vi "Speed Tests 2020-04-08.vi"() -> ()   [LabVIEW 2016]
uses:
  src/Data.ITX/Data.ITX.lvclass
panel:
  in  "Path":path=path "C:/temp"
  out "Another File Size":cluster{i32[], dbl[]}[](graph)=[{[0, 1, 2, 3, 4], [37.234652, 38.890539, 13.243471, 13.252304, 0.0]}, {[0, 1, 2, 3, 4], [37.234652, 38.890539, 13.243471, 13.252304, 0.0]}, {[0, 1, 2, 3, 4], [37.234652, 38.890539, 13.243471, 13.252304, 0.0]}, {[0, 1, 2, 3, 4], [37.234652, 38.890539, 13.243471, 13.252304, 0.0]}, {[0, 1, 2, 3, 4], [37.234652, 38.890539, 13.243471, 13.252304, 0.0]}, {[0, 1, 2, 3, 4], [37.234652, 38.890539, 13.243471, 13.252304, 0.0]}, {[0, 1, 2, 3, 4], [37.234652, 38.890539, 13.243471, 13.252304, 0.0]}, {[0, 1, 2, 3, 4], [37.234652, 38.890539, 13.243471, 13.252304, 0.0]}, {[0, 1, 2, 3, 4], [37.234652, 38.890539, 13.243471, 13.252304, 0.0]}, {[0, 1, 2, 3, 4], [37.234652, 38.890539, 13.243471, 13.252304, 0.0]}, {[0, 1, 2, 3, 4], [37.234652, 38.890539, 13.243471, 13.252304, 0.0]}, {[0, 1, 2, 3, 4], [37.234652, 38.890539, 13.243471, 13.252304, 0.0]}, {[0, 1, 2, 3, 4], [37.234652, 38.890539, 13.243471, 13.252304, 0.0]}, {[0, 1, 2, 3, 4], [37.234652, 38.890539, 13.243471, 13.252304, 0.0]}, {[0, 1, 2, 3, 4], [37.234652, 38.890539, 13.243471, 13.252304, 0.0]}, {[0, 1, 2, 3, 4], [37.234652, 38.890539, 13.243471, 13.252304, 0.0]}, {[0, 1, 2, 3, 4], [37.234652, 38.890539, 13.243471, 13.252304, 0.0]}, {[0, 1, 2, 3, 4], [37.234652, 38.890539, 13.243471, 13.252304, 0.0]}, {[0, 1, 2, 3, 4], [37.234652, 38.890539, 13.243471, 13.252304, 0.0]}, {[0, 1, 2, 3, 4], [37.234652, 38.890539, 13.243471, 13.252304, 0.0]}, {[0, 1, 2, 3, 4], [37.234652, 38.890539, 13.243471, 13.252304, 0.0]}, {[0, 1, 2, 3, 4], [37.234652, 38.890539, 13.243471, 13.252304, 0.0]}, {[0, 1, 2, 3, 4], [37.234652, 38.890539, 13.243471, 13.252304, 0.0]}, {[0, 1, 2, 3, 4], [37.234652, 38.890539, 13.243471, 13.252304, 0.0]}, {[0, 1, 2, 3, 4], [37.234652, 38.890539, 13.243471, 13.252304, 0.0]}, {[0, 1, 2, 3, 4], [37.234652, 38.890539, 13.243471, 13.252304, 0.0]}, {[0, 1, 2, 3, 4], [37.234652, 38.890539, 13.243471, 13.252304, 0.0]}, {[0, 1, 2, 3, 4], [37.234652, 38.890539, 13.243471, 13.252304, 0.0]}, {[0, 1, 2, 3, 4], [37.234652, 38.890539, 13.243471, 13.252304, 0.0]}, {[0, 1, 2, 3, 4], [37.234652, 38.890539, 13.243471, 13.252304, 0.0]}, {[0, 1, 2, 3, 4], [37.234652, 38.890539, 13.243471, 13.252304, 0.0]}, {[0, 1, 2, 3, 4], [37.234652, 38.890539, 13.243471, 13.252304, 0.0]}, {[0, 1, 2, 3, 4], [37.234652, 38.890539, 13.243471, 13.252304, 0.0]}, {[0, 1, 2, 3, 4], [37.234652, 38.890539, 13.243471, 13.252304, 0.0]}, {[0, 1, 2, 3, 4], [37.234652, 38.890539, 13.243471, 13.252304, 0.0]}, {[0, 1, 2, 3, 4], [37.234652, 38.890539, 13.243471, 13.252304, 0.0]}, {[0, 1, 2, 3, 4], [37.234652, 38.890539, 13.243471, 13.252304, 0.0]}]
  out "Read Speed":cluster{i32[], u32[]}[](graph)=[{[0, 1, 2, 3, 4], [1571, 362, 78, 30, 279]}, {[0, 1, 2, 3, 4], [1438, 412, 84, 27, 279]}, {[0, 1, 2, 3, 4], [1431, 378, 71, 25, 279]}, {[0, 1, 2, 3, 4], [1332, 340, 109, 26, 279]}, {[0, 1, 2, 3, 4], [1312, 344, 64, 25, 279]}, {[0, 1, 2, 3, 4], [1361, 338, 132, 38, 279]}, {[0, 1, 2, 3, 4], [1358, 385, 88, 22, 279]}, {[0, 1, 2, 3, 4], [1333, 346, 70, 26, 279]}, {[0, 1, 2, 3, 4], [1332, 346, 67, 29, 279]}, {[0, 1, 2, 3, 4], [1364, 352, 65, 26, 279]}, {[0, 1, 2, 3, 4], [1322, 339, 72, 30, 279]}, {[0, 1, 2, 3, 4], [1363, 352, 68, 31, 279]}, {[0, 1, 2, 3, 4], [1354, 343, 118, 25, 279]}, {[0, 1, 2, 3, 4], [1409, 372, 69, 30, 279]}, {[0, 1, 2, 3, 4], [1423, 403, 71, 26, 279]}, {[0, 1, 2, 3, 4], [1354, 341, 67, 27, 279]}, {[0, 1, 2, 3, 4], [1316, 338, 70, 27, 279]}, {[0, 1, 2, 3, 4], [1353, 365, 67, 27, 279]}, {[0, 1, 2, 3, 4], [1370, 324, 114, 28, 279]}, {[0, 1, 2, 3, 4], [1411, 368, 65, 28, 279]}, {[0, 1, 2, 3, 4], [1355, 349, 115, 27, 279]}, {[0, 1, 2, 3, 4], [1302, 369, 64, 27, 279]}, {[0, 1, 2, 3, 4], [1398, 350, 73, 22, 279]}, {[0, 1, 2, 3, 4], [1344, 361, 64, 29, 279]}, {[0, 1, 2, 3, 4], [1340, 336, 66, 30, 279]}, {[0, 1, 2, 3, 4], [1366, 339, 64, 28, 279]}, {[0, 1, 2, 3, 4], [1386, 358, 178, 33, 279]}, {[0, 1, 2, 3, 4], [1361, 349, 65, 29, 279]}, {[0, 1, 2, 3, 4], [1375, 338, 66, 26, 279]}, {[0, 1, 2, 3, 4], [1332, 365, 65, 26, 279]}, {[0, 1, 2, 3, 4], [1371, 367, 67, 27, 279]}, {[0, 1, 2, 3, 4], [1363, 358, 68, 28, 279]}, {[0, 1, 2, 3, 4], [1493, 354, 66, 29, 279]}, {[0, 1, 2, 3, 4], [1344, 364, 68, 30, 279]}, {[0, 1, 2, 3, 4], [1365, 356, 123, 26, 279]}, {[0, 1, 2, 3, 4], [1348, 355, 66, 31, 279]}, {[0, 1, 2, 3, 4], [1397, 346, 66, 28, 279]}]
  out "Write Speed":cluster{i32[], u32[]}[](graph)=[{[0, 1, 2, 3, 4], [3526, 2046, 105, 42, 2323]}, {[0, 1, 2, 3, 4], [3150, 1985, 87, 39, 2323]}, {[0, 1, 2, 3, 4], [3184, 2046, 84, 37, 2323]}, {[0, 1, 2, 3, 4], [3311, 1954, 99, 36, 2323]}, {[0, 1, 2, 3, 4], [3164, 2044, 101, 35, 2323]}, {[0, 1, 2, 3, 4], [3134, 2044, 79, 34, 2323]}, {[0, 1, 2, 3, 4], [3111, 2010, 78, 35, 2323]}, {[0, 1, 2, 3, 4], [3186, 2036, 81, 35, 2323]}, {[0, 1, 2, 3, 4], [3107, 1993, 82, 39, 2323]}, {[0, 1, 2, 3, 4], [3131, 1956, 80, 35, 2323]}, {[0, 1, 2, 3, 4], [3094, 1935, 85, 31, 2323]}, {[0, 1, 2, 3, 4], [3091, 1982, 86, 36, 2323]}, {[0, 1, 2, 3, 4], [3121, 2010, 87, 35, 2323]}, {[0, 1, 2, 3, 4], [3167, 2007, 83, 33, 2323]}, {[0, 1, 2, 3, 4], [3131, 2006, 80, 33, 2323]}, {[0, 1, 2, 3, 4], [3361, 1961, 82, 35, 2323]}, {[0, 1, 2, 3, 4], [3141, 1961, 82, 37, 2323]}, {[0, 1, 2, 3, 4], [3127, 1976, 79, 38, 2323]}, {[0, 1, 2, 3, 4], [3109, 1931, 81, 36, 2323]}, {[0, 1, 2, 3, 4], [3109, 1963, 80, 34, 2323]}, {[0, 1, 2, 3, 4], [3138, 1964, 81, 35, 2323]}, {[0, 1, 2, 3, 4], [3096, 1997, 82, 32, 2323]}, {[0, 1, 2, 3, 4], [3174, 2025, 82, 36, 2323]}, {[0, 1, 2, 3, 4], [3150, 1948, 80, 34, 2323]}, {[0, 1, 2, 3, 4], [3103, 2020, 83, 36, 2323]}, {[0, 1, 2, 3, 4], [3093, 1953, 82, 33, 2323]}, {[0, 1, 2, 3, 4], [3154, 2010, 83, 39, 2323]}, {[0, 1, 2, 3, 4], [3143, 1997, 79, 33, 2323]}, {[0, 1, 2, 3, 4], [3098, 1988, 85, 35, 2323]}, {[0, 1, 2, 3, 4], [3096, 1950, 80, 36, 2323]}, {[0, 1, 2, 3, 4], [3165, 2000, 77, 32, 2323]}, {[0, 1, 2, 3, 4], [3186, 1989, 79, 41, 2323]}, {[0, 1, 2, 3, 4], [3154, 2153, 80, 35, 2323]}, {[0, 1, 2, 3, 4], [3141, 1998, 87, 35, 2323]}, {[0, 1, 2, 3, 4], [3156, 2030, 81, 37, 2323]}, {[0, 1, 2, 3, 4], [3127, 1989, 80, 33, 2323]}, {[0, 1, 2, 3, 4], [3084, 2012, 80, 34, 2323]}]
  # "DAT"
  # "ITX"
  # "TDMS"
  # "HDF5"
  # "VI"
  # "DAT"
  # "ITX"
  # "TDMS"
  # "HDF5"
  # "VI"
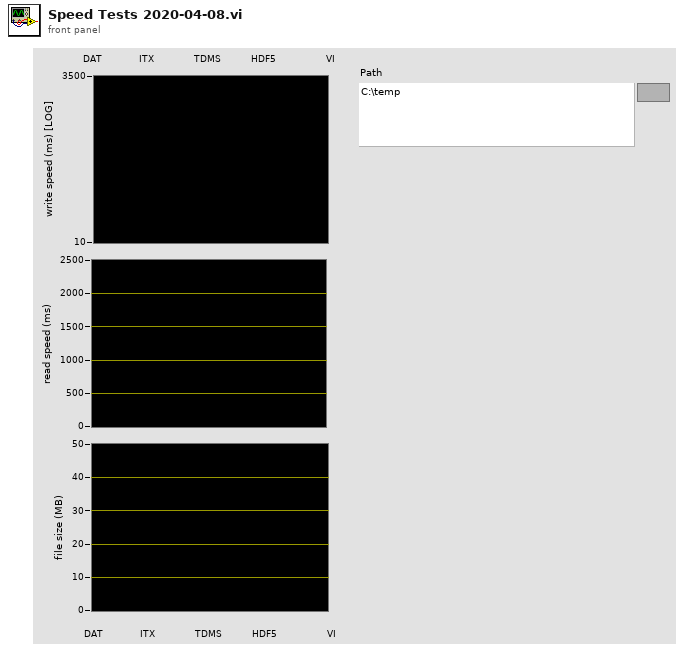
[diagram p1: front panel]
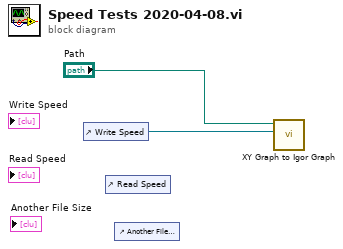
[diagram p0: block diagram]
diagram:
  n1 = control-ref of="Write Speed"() -> (w1:refnum<vi>)
  n2 = control-ref of="Read Speed"() -> ()  [unwired: 1 out]
  n3 = control-ref of="Another File Size"() -> ()  [unwired: 1 out]
  n4 = call "XY Graph to Igor Graph.vi"("XY Graph Reference"=w1, "Path"="Path") -> ()  [unwired: 8 in, 2 out]
